vi "Destroy Buffer.vi"(8 "error in (no error)":errorcluster, 11 "2D U16 DVR Array in":refnum<class "2D U16 DVR Array.lvclass">) -> (0 "error out":errorcluster, 3 "2D U16 DVR Array out":refnum<class "2D U16 DVR Array.lvclass">)   [LabVIEW 2024, in "2D U16 DVR Array.lvclass"]
uses:
  2D U16 DVR Array.lvclass
  2D U16 DVR Array.lvclass/2D U16 DVR Array.ctl
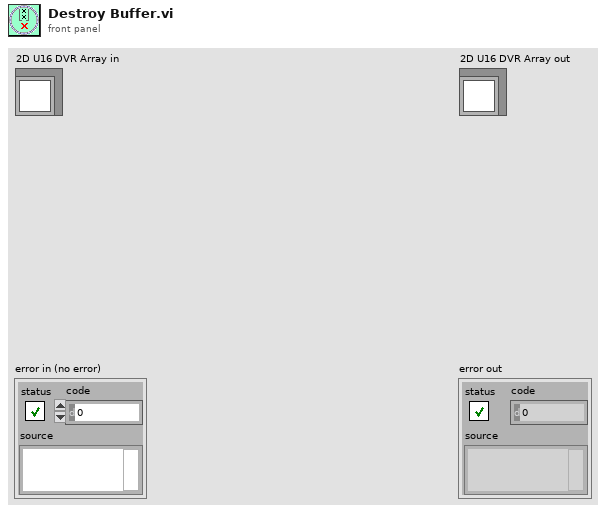
[diagram p1: front panel]
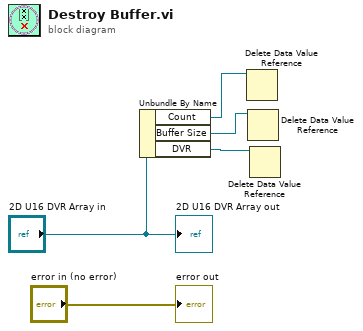
[diagram p0: block diagram]
diagram:
  n1 = Unbundle By Name("2D U16 DVR Array in") -> ("Count"=w1:refnum<data-value>, "Buffer Size"=w2:refnum<data-value>, "DVR"=w3:refnum<data-value>)
  n2 = Delete Data Value Reference(data value reference=w1) -> ()  [unwired: 1 in, 2 out]
  n3 = Delete Data Value Reference(data value reference=w2) -> ()  [unwired: 1 in, 2 out]
  n4 = Delete Data Value Reference(data value reference=w3) -> ()  [unwired: 1 in, 2 out]
  "error out" <- "error in (no error)"
  "2D U16 DVR Array out" <- "2D U16 DVR Array in"
